vi "Read ConfigFilePath.vi"(8 "error in (no error)":errorcluster, 11 "Config in":refnum<class "Config.lvclass">) -> (0 "error out":errorcluster, 2 "ConfigFilePath":path, 3 "Config out":refnum<class "Config.lvclass">)   [LabVIEW 2014, in "Framework.lvlib" / "Config.lvclass"]
uses:
  Config.lvclass
  Config.lvclass/Config.ctl
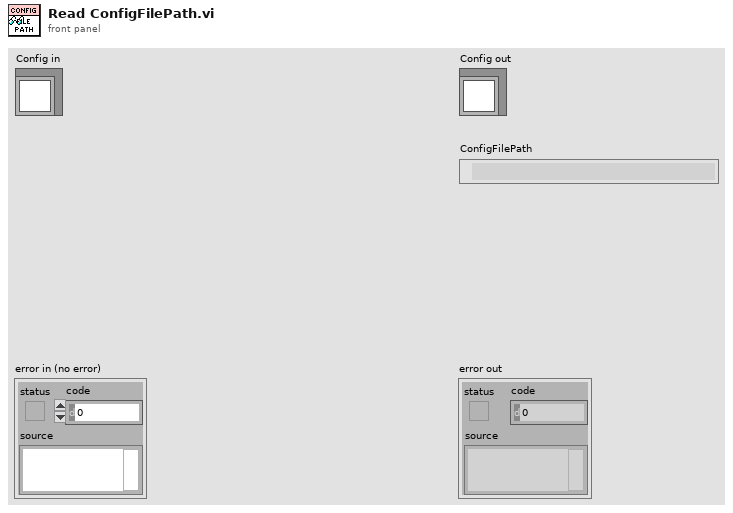
[diagram p1: front panel]
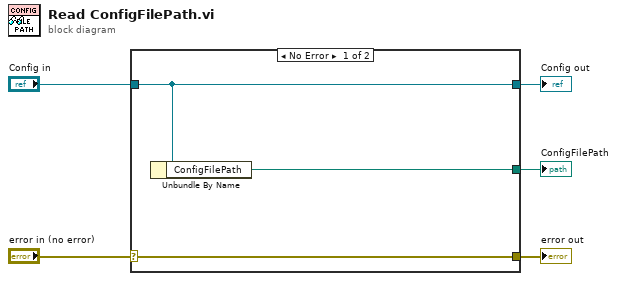
[diagram p0: block diagram]
diagram:
  n1 = case shown="No Error" "error in (no error)" {
    selector: "error in (no error)" -> [w8 w9]
    tunnel: [w8 w9] -> w4
    tunnel: [w7 w10] -> w2
    tunnel: "Config in" -> [w7 w10]
    tunnel: [w6 _] -> w1
    frame No Error {
      n2 = Unbundle By Name(w7) -> ("ConfigFilePath"=w6:path)
    }
    frame Error {
    }
  }
  "error out" <- w4
  "Config out" <- w2
  "ConfigFilePath" <- w1
